vi "Configure Spectral (Phase).vi"(0 "VISA resource name":refnum<visa-resource-name>, 1 "Frequency Span (100kHz)":dbl=100000.0, 2 "Resolution BW (400Hz)":dbl=400000.0, 3 "Gate Position (0s)":dbl, 5 "Channel (4:Math1)":u16(ring)=4 items=["Math1"=4, "Math2"=5, "Math3"=6, "Math4"=7], 7 "Scale (0:Degrees)":u16(ring) items=["Degrees", "Radians", "Groupdelay"], 11 "error in (no error)":errorcluster, 12 "Suppression Threshold (-200dB)":dbl=-200.0, 13 "Unwrap (OFF)":bool caption="Unwrap", 14 "Window Type (0:Rectangular)":u16(ring) items=["Rectangular", "Hamming", "Hanning", "KaiserBessel", "Black-Harris", "Flattop2", "Gaussian", "TekExp"]) -> (4 "VISA resource name out":refnum<visa-resource-name>, 15 "error out":errorcluster)   [LabVIEW 2011, in "Tektronix 7000 Series.lvlib"]
doc: "Configures the spectral phase for a specified mathematical waveform."
uses:
  Tektronix 7000 Series.lvlib
panel:
  # "Basic Configure"
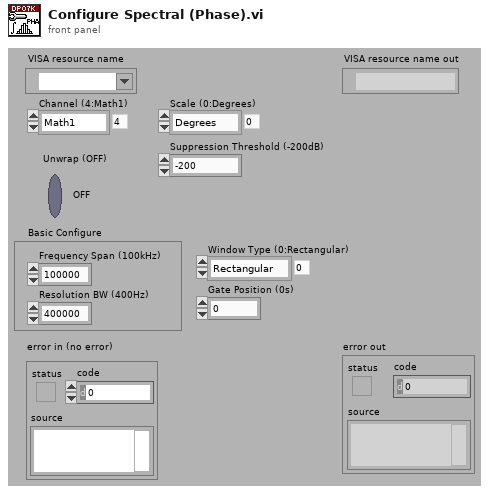
[diagram p1: front panel]
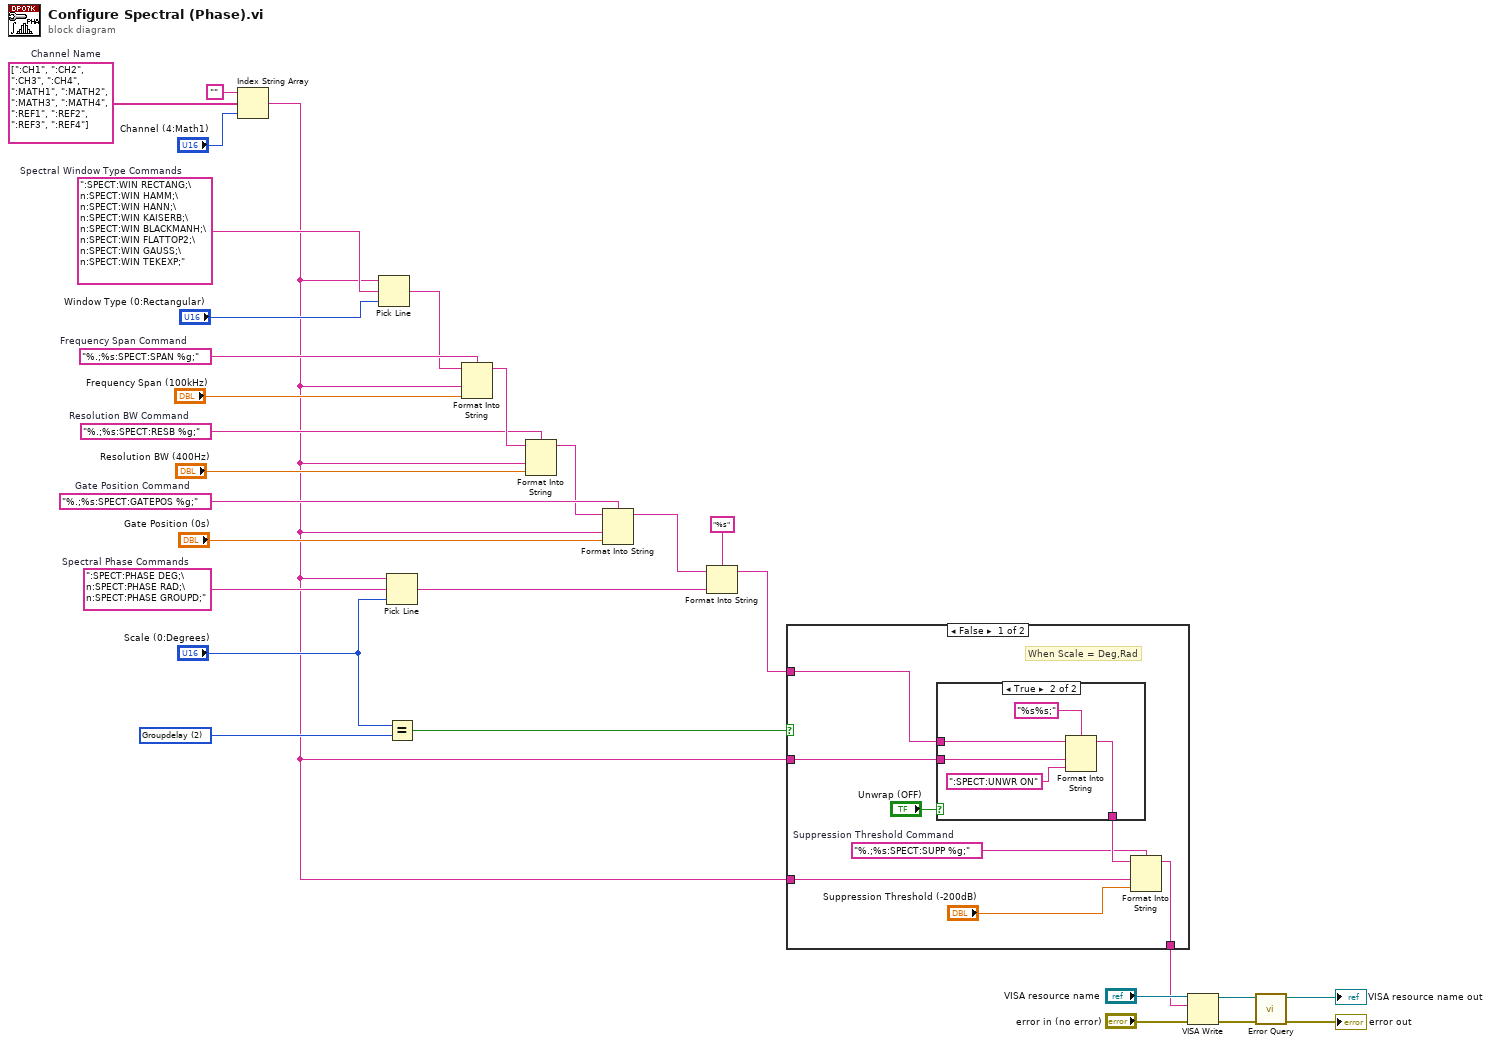
[diagram p0: block diagram]
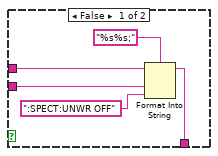
[diagram p2: hidden frame]
diagram:
  w17 = "%.;%s:SPECT:GATEPOS %g;"  # Gate Position Command
  w18 = ":SPECT:WIN RECTANG;\n:SPECT:WIN HAMM;\n:SPECT:WIN HANN;\n:SPECT:WIN KAISERB;\n:SPECT:WIN BLACKMANH;\n:SPECT:WIN FLATTOP2;\n:SPECT:WIN GAUSS;\n:SPECT:WIN TEKEXP;"  # Spectral Window Type Commands
  w19 = "%.;%s:SPECT:RESB %g;"  # Resolution BW Command
  w22 = "%.;%s:SPECT:SPAN %g;"  # Frequency Span Command
  w25 = u16 2 items=["Degrees", "Radians", "Groupdelay"] ("Scale(0:Degrees)")
  w29 = string[] [":CH1", ":CH2", ":CH3", ":CH4", ":MATH1", ":MATH2", ":MATH3", ":MATH4", ":REF1", ":REF2", ":REF3", ":REF4"]  # Channel Name
  w27 = ":SPECT:PHASE DEG;\n:SPECT:PHASE RAD;\n:SPECT:PHASE GROUPD;"  # Spectral Phase Commands
  n1 = Index String Array(1:"Channel (4:Math1)", 2:w29, 3:"") -> (0:w3:string)
  n2 = Pick Line(string ("")=w3, multi-line string=w18, line index="Window Type (0:Rectangular)") -> (output string=w2:string)
  n3 = Pick Line(string ("")=w3, multi-line string=w27, line index="Scale (0:Degrees)") -> (output string=w7:string)
  n4 = Equal?(x="Scale (0:Degrees)", y=w25) -> (x = y?=w24:bool)
  n5 = Format Into String(format string=w22, initial string=w2, w3, "Frequency Span (100kHz)") -> (resulting string=w21:string)  [unwired: 1 in, 1 out]
  n6 = Format Into String(format string=w19, initial string=w21, w3, "Resolution BW (400Hz)") -> (resulting string=w1:string)  [unwired: 1 in, 1 out]
  n7 = Format Into String(format string=w17, initial string=w1, w3, "Gate Position (0s)") -> (resulting string=w6:string)  [unwired: 1 in, 1 out]
  n8 = Format Into String(format string="%s", initial string=w6, w7) -> (resulting string=w8:string)  [unwired: 1 in, 1 out]
  n9 = case shown="False" w24 {
    tunnel: w8 -> [w36 w49]
    tunnel: w3 -> [w37 _]
    tunnel: w3 -> [w32 _]
    tunnel: [w31 w49] -> w10
    frame False {
      w34 = "%.;%s:SPECT:SUPP %g;"  # Suppression Threshold Command
      # "When Scale = Deg,Rad"
      n10 = case shown="True" "Unwrap (OFF)" {
        tunnel: w37 -> [w40 w48]
        tunnel: w36 -> [w41 w46]
        tunnel: [w39 w44] -> w35
        frame False {
          n11 = Format Into String(format string="%s%s;", initial string=w41, w40, ":SPECT:UNWR OFF" ("input 2")) -> (resulting string=w39:string)  [unwired: 1 in, 1 out]
        }
        frame True {
          n12 = Format Into String(format string="%s%s;", initial string=w46, w48, ":SPECT:UNWR ON" ("input 2")) -> (resulting string=w44:string)  [unwired: 1 in, 1 out]
        }
      }
      n13 = Format Into String(format string=w34, initial string=w35, w32, "Suppression Threshold (-200dB)") -> (resulting string=w31:string)  [unwired: 1 in, 1 out]
    }
    frame True {
    }
  }
  n14 = VISA Write(VISA resource name="VISA resource name", write buffer=w10, error in (no error)="error in (no error)") -> (VISA resource name out=w15:refnum<visa-resource-name>, error out=w16:errorcluster)  [unwired: 1 out]
  n15 = call "Error Query.vi"("error in (no error)"=w16, "VISA resource name"=w15) -> ("error out"=→"error out":errorcluster, "VISA resource name out"=→"VISA resource name out":refnum<visa-resource-name>)  [unwired: 6 in, 2 out]
